vi "PreProcess.vi"(8 "error in (no error)":errorcluster, 10 "Variant in":variant, 11 "ONNX Angle Class in":refnum<class "ONNX Angle Class.lvclass">) -> (0 "error out":errorcluster, 2 "Variant out":variant, 3 "ONNX Angle Class out":refnum<class "ONNX Angle Class.lvclass">)   [LabVIEW 2017, in "ONNX Angle Class Library.lvlib" / "ONNX Angle Class.lvclass"]
uses:
  ONNX Angle Class.lvclass
  ONNX Angle Class.lvclass/ONNX Angle Class.ctl
  <vilib>/picture/picture.llb/imagedata.ctl
  ONNX YOLO Class/TypeDef/Circle.ctl
  ONNX YOLO Class/ONNX YOLO Class Library.lvlib
  ONNX Angle Class Library.lvlib
panel:
  out "picture":picture
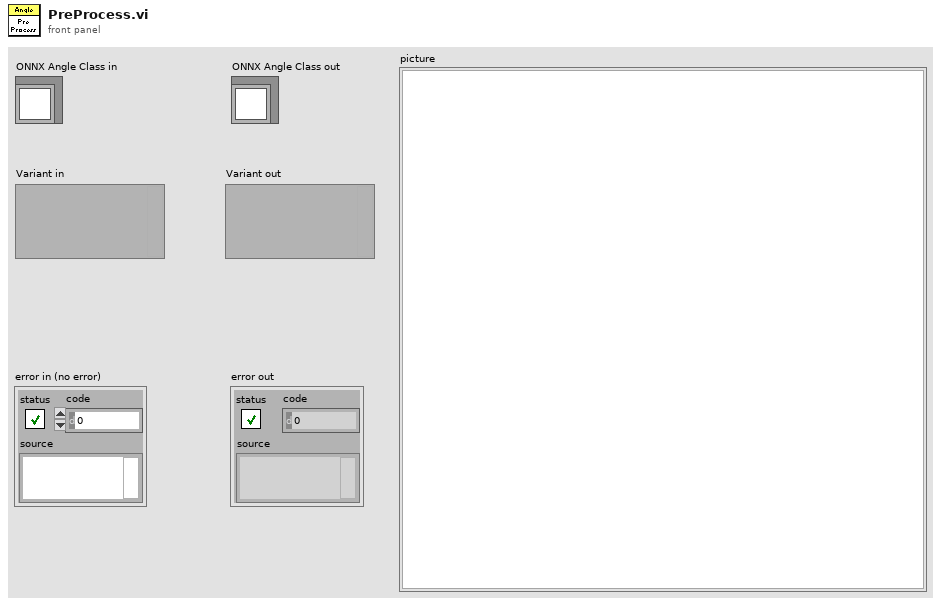
[diagram p1: front panel]
types:
  T1 = typedef "imagedata.ctl" = cluster{"image type":i32, "image depth":i32, "image":u8[], "mask":u8[], "colors":u32[], "Rectangle":cluster{"left":i16, "top":i16, "right":i16, "bottom":i16}}
  T2 = typedef "ONNX YOLO Class Library.lvlib/Circle.ctl" = cluster{"x":sgl, "y":sgl, "r":sgl}
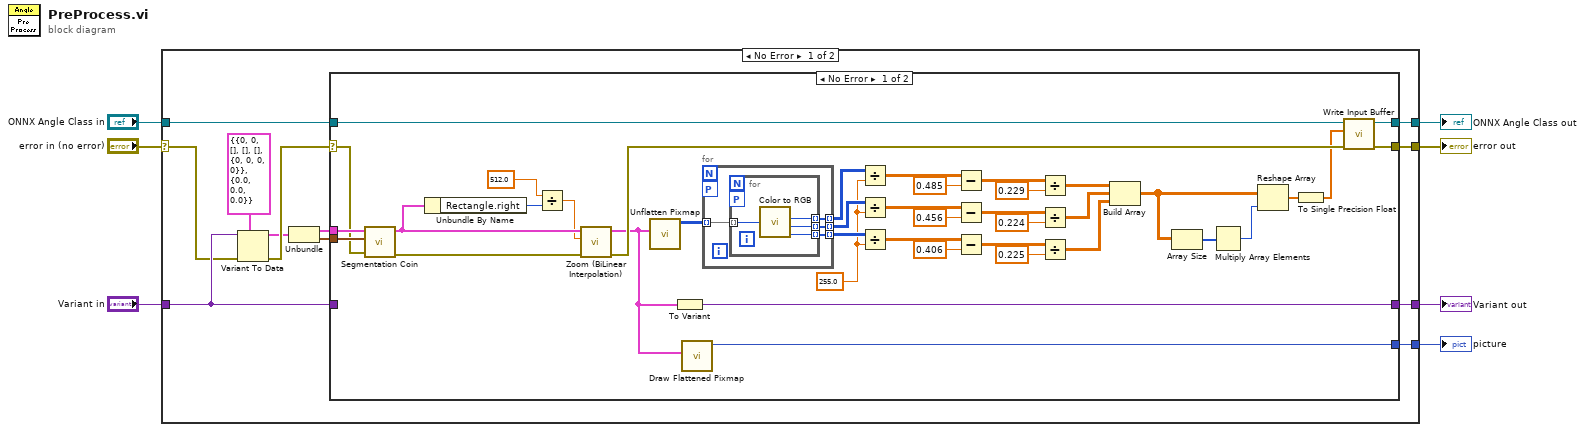
[diagram p0: block diagram]
diagram:
  n1 = case shown="No Error" "error in (no error)" {
    selector: "error in (no error)" -> [w12 w72]
    tunnel: "ONNX Angle Class in" -> [w17 w73]
    tunnel: [w16 w73] -> w6
    tunnel: [w15 w72] -> w2
    tunnel: "Variant in" -> [w14 w71]
    tunnel: [w13 w71] -> w4
    tunnel: [w8 _] -> w1
    frame No Error {
      n2 = Variant To Data(error in=w12, type=cluster{"image data":T1, "Circle":T2} {"image data"={"image type"=0, "image depth"=0, "image"=[], "mask"=[], "colors"=[], "Rectangle"={"left"=0, "top"=0, "right"=0, "bottom"=0}}, "Circle"={"x"=0.0, "y"=0.0, "r"=0.0}} ("output cluster"), Variant=w14) -> (data=w18:cluster{"image data":T1, "Circle":T2}, error out=w19:errorcluster)
      n3 = Unbundle(w18) -> ("image data"=w10:T1, "Circle"=w9:T2)
      n4 = case shown="No Error" w19 {
        selector: w19 -> [w49 w69]
        tunnel: w10 -> [w51 _]
        tunnel: w17 -> [w59 w70]
        tunnel: [w58 w70] -> w16
        tunnel: [w57 w69] -> w15
        tunnel: w14 -> [_ w68]
        tunnel: [w47 w68] -> w13
        tunnel: w9 -> [w50 _]
        tunnel: [w46 _] -> w8
        frame No Error {
          w37 = 255.0 ("y")
          n5 = call "Segmentation Coin.vi"("error in (no error)"=w49, "Circle"=w50, "image data in"=w51) -> ("error out"=w56:errorcluster, "image data out"=w55:T1)  [unwired: 7 in]
          n6 = Unbundle By Name(w55) -> ("Rectangle.right"=w54:i16)
          n7 = Divide(x=512.0, y=w54) -> (x/y=w53:dbl)
          n8 = call "Zoom (BiLinear Interpolation).vi"("error IN"=w56, "Zoom Coefficient"=w53, "image data IN"=w55) -> ("error OUT"=w48:errorcluster, "image data OUT"=w21:T1)  [unwired: 7 in]
          n9 = call <vilib>:"Unflatten Pixmap.vi"("image data"=w21) -> ("24-bit pixmap"=w45:u32[][])  [unwired: 10 out]
          n10 = To Variant(anything=w21) -> (Variant=w47:variant)
          n11 = call <vilib>:"Draw Flattened Pixmap.vi"("image data"=w21) -> ("new picture"=w46:picture)  [unwired: 8 in]
          n12 = for {
            tunnel: w45 -> [w63] mode=indexing
            tunnel: [w62] -> w38 mode=indexing
            tunnel: [w61] -> w39 mode=indexing
            tunnel: [w60] -> w40 mode=indexing
            workers-P: _ -> [_]
            n13 = for {
              tunnel: w63 -> [w64] mode=indexing
              tunnel: [w67] -> w62 mode=indexing
              tunnel: [w66] -> w61 mode=indexing
              tunnel: [w65] -> w60 mode=indexing
              workers-P: _ -> [_]
              n14 = call <vilib>:"Color to RGB.vi"("Color"=w64) -> ("R"=w67:u8, "G"=w66:u8, "B"=w65:u8)  [unwired: 1 out]
            }
          }
          n15 = Divide(x=w38, y=w37) -> (x/y=w36:dbl[][])
          n16 = Divide(x=w39, y=w37) -> (x/y=w25:dbl[][])
          n17 = Divide(x=w40, y=w37) -> (x/y=w23:dbl[][])
          n18 = Subtract(x=w36, y=0.485) -> (x-y=w34:dbl[][])
          n19 = Subtract(x=w25, y=0.456) -> (x-y=w26:dbl[][])
          n20 = Subtract(x=w23, y=0.406) -> (x-y=w28:dbl[][])
          n21 = Divide(x=w34, y=0.229) -> (x/y=w33:dbl[][])
          n22 = Divide(x=w26, y=0.224) -> (x/y=w24:dbl[][])
          n23 = Divide(x=w28, y=0.225) -> (x/y=w22:dbl[][])
          n24 = Build Array(w33, w24, w22) -> (w42:dbl[][][])
          n25 = Array Size(array=w42) -> (size(s)=w41:i32[])
          n26 = Multiply Array Elements(1:w41) -> (0:w43:i32)
          n27 = Reshape Array(w42, w43) -> (w44:dbl[])
          n28 = To Single Precision Float(number=w44) -> (single precision float=w20:sgl[])
          n29 = call-dynamic "Write Input Buffer.vi"("error in (no error)"=w48, "Input Buffer"=w20, "ONNX Class in"=w59) -> ("error out"=w57:errorcluster, "ONNX Class out"=w58:refnum<class "ONNX Angle Class.lvclass">)  [unwired: 7 in]
        }
        frame Error {
        }
      }
    }
    frame Error {
    }
  }
  "error out" <- w2
  "ONNX Angle Class out" <- w6
  "Variant out" <- w4
  "picture" <- w1
